vi "AlliGator Compute Sliced Mean, SDV & CV Plots.vi"(8 "error in (no error)":errorcluster, 10 "tau(I) Plot":cluster{"X Array":dbl[], "Y Array":dbl[]}, 11 "Slices Definition":T3={"Axis Start"=0.0, "Axis Stop"=0.0, "# Steps"=0, "Step Size"=1.0, "Step Definition"=enum."# Steps", "Upper Percentile"=1.0, "Lower Percentile"=1.0, "Min # Data Points/Slice"=1, "Output Abscissa Statistics Plots"=FALSE, "Bin Location"=enum."Left", "# Elements"=1, "Bootstrap CV's SDV"=FALSE, "# Replicas"=1} {"# Replicas" min=1; "# Elements" min=0; "Min # Data Points/Slice" min=0 max=100; "Lower Percentile" min=0.0 max=100.0; "Upper Percentile" min=0.0 max=100.0; "Step Size" min=1.0; "# Steps" min=1}) -> (0 "error out":errorcluster, 1 "Bootstrap CV's SDV":bool, 2 "Bin Intensity Distribution (unused)":cluster{"Intensity Array":sgl[]}[](array[cluster]), 3 "Result Plots Cluster":T1)   [LabVIEW 2021, in "AlliGator Lifetime & Other Parameters.lvlib"]
doc: "Computes sliced data statistics."
uses:
  AlliGator Lifetime & Other Parameters.lvlib
  Graphs/XY Graph/XY Graph Sliced Mean & SDV Step Definition.ctl
  AlliGator Intensity Slice Definition.ctl
  Graphs/XY Graph/XY Graph Sliced CV Abscissa Location.ctl
  Decay Fit Parameter Map/AlliGator Sliced Analysis Plots.ctl
  Graphs/XY Graph/XY Graph Plot Data.ctl
  f27c31c8-11a2-4adc-8bf5-3f0847906007.vi
  e52038b9-098e-46eb-bc49-b571e133bb6c.vi
  <userlib>/_OpenG.lib/array/array.llb/Sort 1D Array (DBL)__ogtk.vi
  <vilib>/gmath/statdist.llb/st_Percentiles (array).vi
  <vilib>/Utility/error.llb/Error Cluster From Error Code.vi
  <userlib>/_OpenG.lib/array/array.llb/openg_array.lvlib
  <vilib>/gmath/NI_Gmath.lvlib
  Error/Error.lvlib
  Graphs/XY Graph/XY Graph Add-Ons.lvlib
  Decay Fit Parameter Map/AlliGator Decay Fit Parameter Map.lvlib
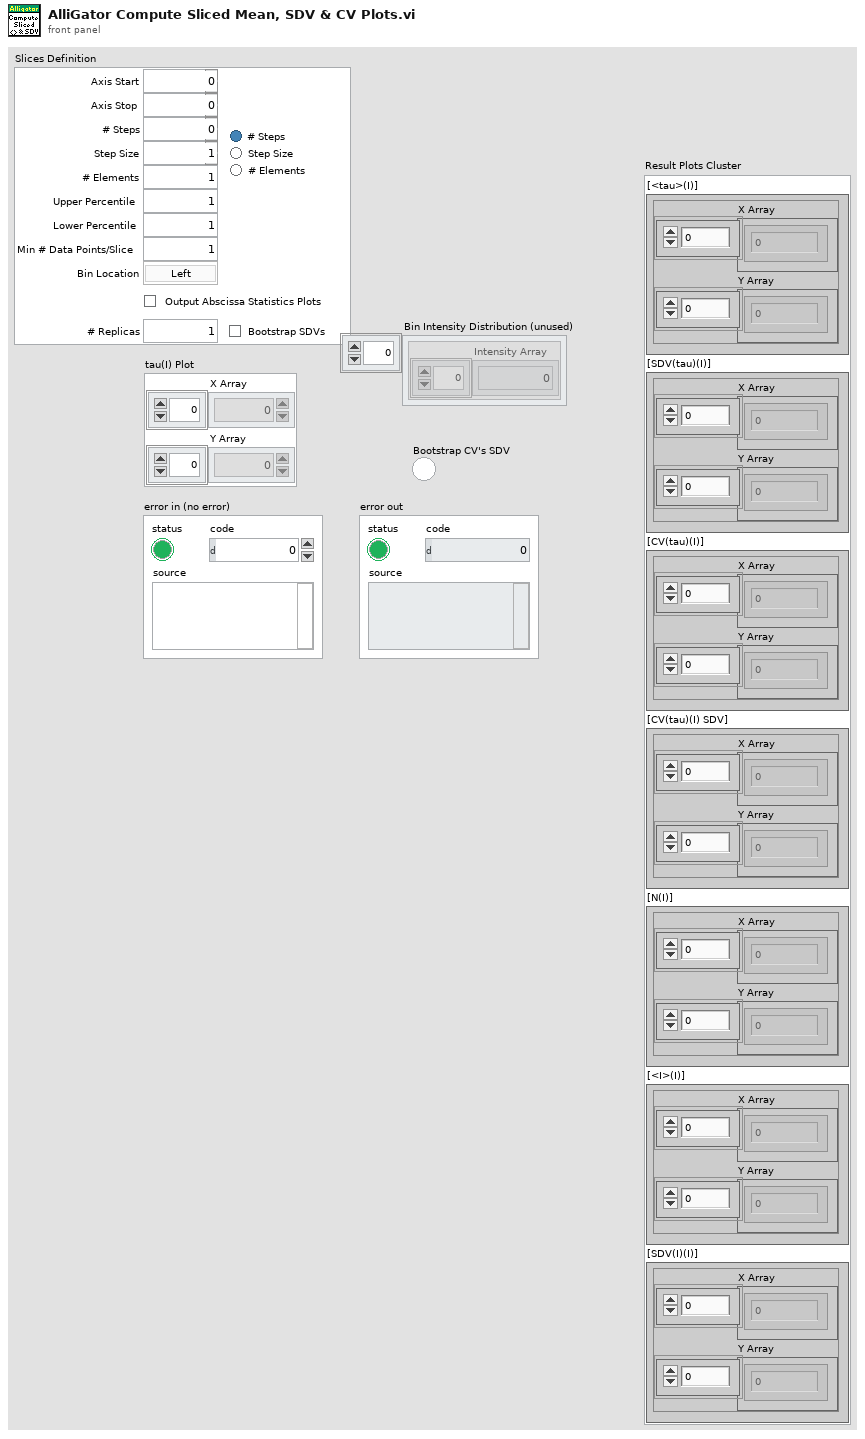
[diagram p1: front panel]
types:
  T1 = typedef "AlliGator Decay Fit Parameter Map.lvlib/AlliGator Sliced Analysis Plots.ctl" = cluster{"[<tau>(I)]":T2, "[SDV(tau)(I)]":T2, "[CV(tau)(I)]":T2, "[CV(tau)(I) SDV]":T2, "[N(I)]":T2, "[<I>(I)]":T2, "[SDV(I)(I)]":T2}
  T2 = typedef "XY Graph Add-Ons.lvlib/XY Graph Plot Data.ctl" = cluster{"X Array":dbl[], "Y Array":dbl[]}
  T3 = typedef "XY Graph Add-Ons.lvlib/XY Graph Sliced Mean & SDV Step Definition.ctl" = cluster{"Axis Start":dbl, "Axis Stop":dbl, "# Steps":i32, "Step Size":dbl, "Step Definition":T4, "Upper Percentile":dbl, "Lower Percentile":dbl, "Min # Data Points/Slice":i32, "Output Abscissa Statistics Plots":bool, "Bin Location":T5, "# Elements":i32, "Bootstrap CV's SDV":bool, "# Replicas":i32}
  T4 = typedef "AlliGator Lifetime & Other Parameters.lvlib/AlliGator Intensity Slice Definition.ctl" = enum32{"# Steps", "Step Size", "# Elements"}
  T5 = typedef "XY Graph Add-Ons.lvlib/XY Graph Sliced CV Abscissa Location.ctl" = enum16{"Left", "Center", "Mean", "Right"}
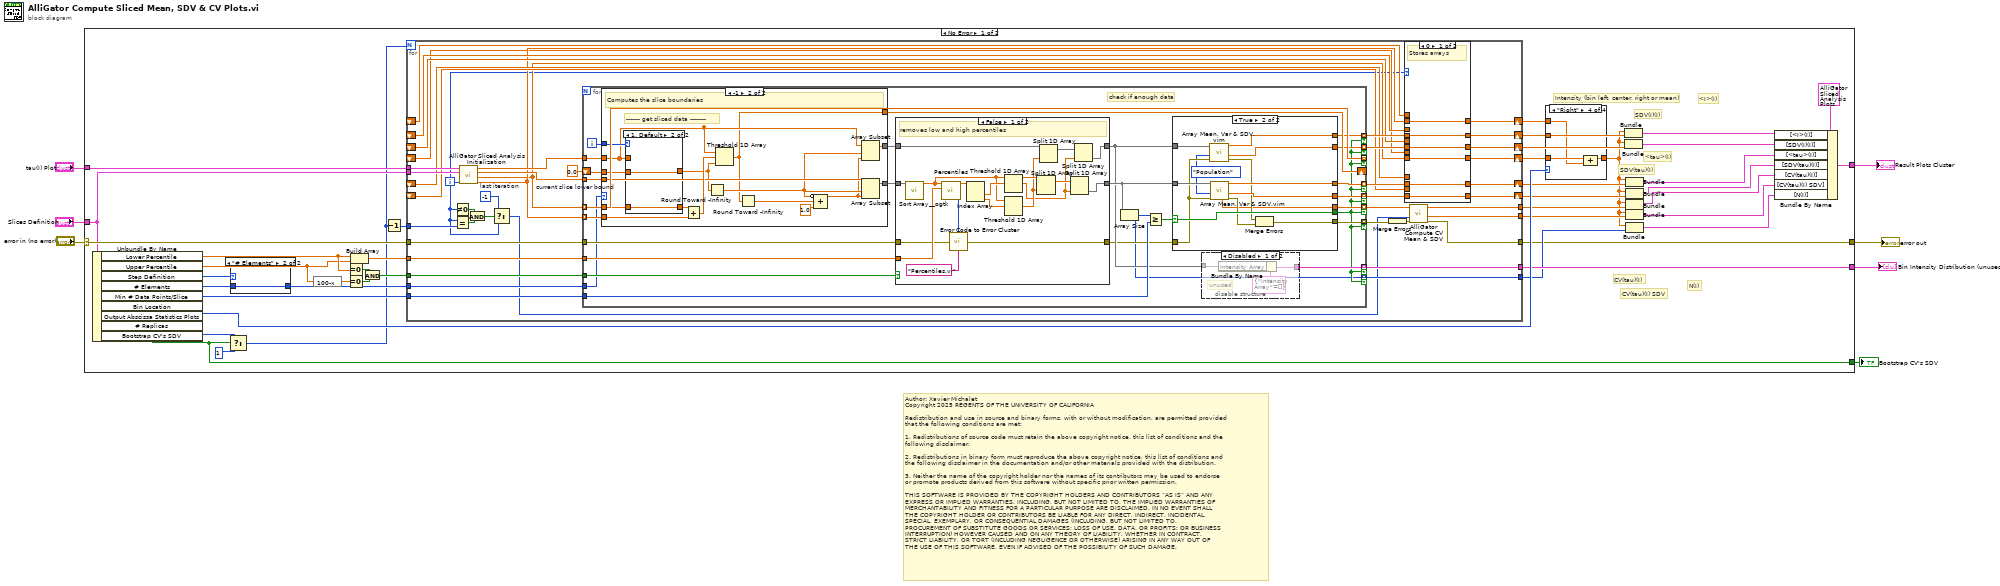
[diagram p0: block diagram]
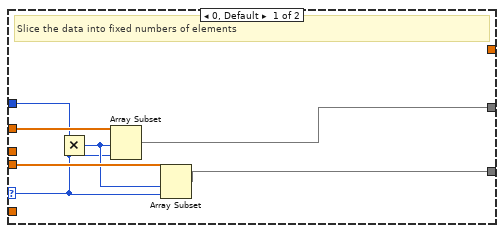
[diagram p5: hidden frame]
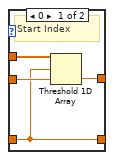
[diagram p6: hidden frame]
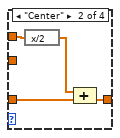
[diagram p9: hidden frame]
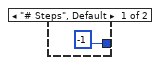
[diagram p11: hidden frame]
diagram:
  # "Author: Xavier Michalet\nCopyright 2025 REGENTS OF THE UNIVERSITY OF CALIFORNIA\n\nRedistribution and use in source and binary forms, with or without modification, are permitted provided\nthat the following conditions are met:\n\n1. Redistributions of source code must retain the above copyright notice, this list of conditions and the\nfollowing disclaimer.\n\n2. Redistributions in binary form must reproduce the above copyright notice, this list of conditions and\nthe following disclaimer in the documentation and/or other materials provided with the distribution.\n\n3. Neither the name of the copyright holder nor the names of its contributors may be used to endorse \nor promote products derived from this software without specific prior written permission.\n\nTHIS SOFTWARE IS PROVIDED BY THE COPYRIGHT HOLDERS AND CONTRIBUTORS “AS IS” AND ANY \nEXPRESS OR IMPLIED WARRANTIES, INCLUDING, BUT NOT LIMITED TO, THE IMPLIED WARRANTIES OF\nMERCHANTABILITY AND FITNESS FOR A PARTICULAR PURPOSE ARE DISCLAIMED. IN NO EVENT SHALL\nTHE COPYRIGHT HOLDER OR CONTRIBUTORS BE LIABLE FOR ANY DIRECT, INDIRECT, INCIDENTAL, \nSPECIAL, EXEMPLARY, OR CONSEQUENTIAL DAMAGES (INCLUDING, BUT NOT LIMITED TO, \nPROCUREMENT OF SUBSTITUTE GOODS OR SERVICES; LOSS OF USE, DATA, OR PROFITS; OR BUSINESS\nINTERRUPTION) HOWEVER CAUSED AND ON ANY THEORY OF LIABILITY, WHETHER IN CONTRACT, \nSTRICT LIABILITY, OR TORT (INCLUDING NEGLIGENCE OR OTHERWISE) ARISING IN ANY WAY OUT OF\nTHE USE OF THIS SOFTWARE, EVEN IF ADVISED OF THE POSSIBILITY OF SUCH DAMAGE."
  n1 = case shown="No Error" "error in (no error)" {
    selector: "error in (no error)" -> [w36 w207]
    tunnel: "tau(I) Plot" -> [w32 _]
    tunnel: "Slices Definition" -> [w31 _]
    tunnel: [w17 w207] -> w4
    tunnel: [w39 _] -> w3
    tunnel: [w12 _] -> w2
    tunnel: [w10 _] -> w1
    frame No Error {
      # "CV(tau)(I) SDV"
      # "N(I)"
      # "CV(tau)(I)"
      # "SDV(tau)(I)"
      # "<tau>(I)"
      # "SDV(I)(I)"
      # "<I>(I)"
      # "Intensity (bin left, center, right or mean)"
      n2 = Unbundle By Name(w31) -> ("Lower Percentile"=w47:dbl, "Upper Percentile"=w42:dbl, "Step Definition"=w35:T4, "# Elements"=w34:i32, "Min # Data Points/Slice"=w45:i32, "Bin Location"=w40:T5, "# Replicas"=w38:i32, "Bootstrap CV's SDV"=w12:bool)  [unwired: 1 out]
      n3 = Select(t=w38, s=w12, f=1) -> (s? t:f=w9:i32)
      n4 = case shown="\"# Elements\"" w35 {
        tunnel: w34 -> [_ w206]
        tunnel: [-1 ("# Elements") w206] -> w33
        frame "# Steps", Default {
        }
        frame "# Elements" {
        }
      }
      n5 = expression code="100-x"(w42) -> (w41:dbl)
      n6 = Equal To 0?(x=w47) -> (x = 0?=w46:bool)
      n7 = Equal To 0?(x=w41) -> (x = 0?=w44:bool)
      n8 = Build Array(w47, w42) -> (w48:dbl[])
      n9 = And(x=w46, y=w44) -> (x .and. y?=w43:bool)
      n10 = Decrement(x=w9) -> (x-1=w8:i32)
      n11 = for {
        N: w9 -> [_]
        tunnel: [w91] -> w26
        tunnel: w48 -> [w90]
        tunnel: w45 -> [w89]
        tunnel: w43 -> [w88]
        tunnel: [w62] -> w21
        tunnel: [w86] -> w39
        tunnel: [w58] -> w17
        tunnel: w36 -> [w85]
        tunnel: w33 -> [w84]
        tunnel: w32 -> [w83]
        tunnel: w31 -> [w82]
        shift-right: [w77] -> w18
        shift-left: _ -> [w66]
        shift-right: [w75] -> w24
        shift-left: _ -> [w67]
        shift-right: [w74] -> w19
        shift-left: _ -> [w56]
        shift-right: [w72] -> w30
        shift-left: _ -> [w68]
        shift-right: [w70] -> w29
        shift-left: _ -> [w69]
        shift-right: [w64] -> w16
        shift-left: _ -> [w63]
        tunnel: [w61] -> w15
        tunnel: w8 -> [w55]
        i -> [w50]
        w51 = -1  # last iteration
        w79 = 0.0  # current slice lower bound
        n12 = Not Equal To 0?(x=w50) -> (x != 0?=w54:bool)
        n13 = Equal?(x=w50, y=w55) -> (x = y?=w53:bool)
        n14 = call "AlliGator Sliced Analysis Initialization.vi"("Iteration (0)"=w50, "Slices Definition"=w82, "tau(I) Plot"=w83) -> ("[delta I_i]"=w65:dbl[], "[I_i]"=w57:dbl[], "[tau]"=w80:dbl[], "Sorted [I]"=w81:dbl[])  [unwired: 4 in, 1 out]
        n15 = And(x=w54, y=w53) -> (x .and. y?=w52:bool)
        n16 = Select(t=w51, s=w52, f=w50) -> (s? t:f=w49:i32)
        n17 = for {
          tunnel: w57 -> [w121] mode=indexing
          tunnel: w81 -> [w117]
          tunnel: w80 -> [w127]
          shift-right: [w115] -> _
          shift-left: w79 -> [w129]
          tunnel: w65 -> [w128] mode=indexing
          tunnel: [w126] -> w73 mode=indexing if=w107
          tunnel: [w125] -> w71 mode=indexing if=w107
          tunnel: [w104] -> w91 mode=indexing if=w107
          tunnel: w90 -> [w124]
          tunnel: w89 -> [w122]
          tunnel: [w121] -> _ mode=indexing if=w107
          tunnel: w88 -> [w118]
          tunnel: [w114] -> w78 mode=indexing if=w107
          tunnel: [w113] -> w76 mode=indexing if=w107
          tunnel: [w112] -> w87 mode=indexing if=w107
          tunnel: [w110] -> w86 mode=indexing if=w107
          tunnel: [w108] -> w60 mode=indexing if=w107
          tunnel: w85 -> [w106]
          tunnel: w84 -> [w105]
          i -> [w130]
          # "check if enough data"
          n18 = case shown="-1" w105 {
            selector: w105 -> [w165 _]
            tunnel: w130 -> [w169 w186]
            tunnel: w129 -> [_ w185]
            tunnel: w128 -> [_ w183]
            tunnel: w127 -> [w167 w181]
            tunnel: w121 -> [_ w177]
            tunnel: [w164 w176] -> w119
            tunnel: w117 -> [w170 w175]
            tunnel: [w168 w172] -> w116
            tunnel: [_ w171] -> w115
            frame 0, Default {
              # "Slice the data into fixed numbers of elements"
              n19 = Multiply(x=w169, y=w165) -> (x*y=w166:i32)
              n20 = Array Subset(array=w170, index=w166, length=w165) -> (w168:dbl[])
              n21 = Array Subset(array=w167, index=w166, length=w165) -> (w164:dbl[])
            }
            frame -1 {
              # "------- get sliced data --------"
              # "Computes the slice boundaries"
              n22 = case shown="1, Default" w186 {
                tunnel: w175 -> [w190 _]
                tunnel: w177 -> [w187 w192]
                tunnel: w185 -> [w189 w191]
                tunnel: [w188 w191] -> w180
                tunnel: [w187 w192] -> w184
                frame 0 {
                  # "Start Index"
                  n23 = Threshold 1D Array(1:w189, 2:w187, 3:w190) -> (0:w188:dbl)
                }
                frame 1, Default {
                }
              }
              n24 = Add(x=w184, y=w183) -> (x+y=w182:dbl)
              n25 = Round Toward -Infinity(1:w180) -> (0:w174:dbl)
              n26 = Threshold 1D Array(1:w180, 2:w182, 3:w175) -> (0:w171:dbl)
              n27 = Round Toward -Infinity(1:w171) -> (0:w179:dbl)
              n28 = Compound Arithmetic op=ADD(invert w174, w179, 1.0 ("value")) -> (w173:dbl)
              n29 = Array Subset(array=w175, index=w174, length=w173) -> (w172:dbl[])
              n30 = Array Subset(array=w181, index=w174, length=w173) -> (w176:dbl[])
            }
          }
          n31 = case shown="False" w118 {
            tunnel: w124 -> [w161 _]
            tunnel: [w159 w163] -> w123
            tunnel: w119 -> [w155 w163]
            tunnel: w116 -> [w153 w162]
            tunnel: [w150 w162] -> w111
            tunnel: [w146 _] -> w109
            tunnel: w106 -> [w145 _]
            frame False {
              # "removes low and high percentiles"
              n32 = call-poly <userlib>:"Sort Array__ogtk.vi"("Array in"=w155) -> ("Sorted Array out"=w154:dbl[])  [unwired: 9 in, 1 out]
              n33 = call-poly <vilib>:"Percentiles.vi"("p array"=w161, "x array"=w154) -> ("error"=w148:i32, "percentiles"=w160:dbl[])  [unwired: 8 in]
              n34 = call "Error Code to Error Cluster.vi"("Error Code"=w148, "Error Source"="Percentiles.vi", "Error In"=w145) -> ("Error Out"=w146:errorcluster)  [unwired: 12 in]
              n35 = Index Array(array=w160) -> (element #1=w158:dbl, element #2=w156:dbl)  [unwired: 2 in]
              n36 = Threshold 1D Array(2:w158, 3:w154) -> (0:w149:dbl)  [unwired: 1 in]
              n37 = Threshold 1D Array(2:w156, 3:w154) -> (0:w152:dbl)  [unwired: 1 in]
              n38 = Split 1D Array(array=w154, index=w152) -> (first subarray=w157:dbl[])  [unwired: 1 out]
              n39 = Split 1D Array(array=w153, index=w152) -> (first subarray=w151:dbl[])  [unwired: 1 out]
              n40 = Split 1D Array(array=w157, index=w149) -> (second subarray=w159:dbl[])  [unwired: 1 out]
              n41 = Split 1D Array(array=w151, index=w149) -> (second subarray=w150:dbl[])  [unwired: 1 out]
            }
            frame True {
              # "Do not reject outliers"
            }
          }
          n42 = Array Size(array=w123) -> (size(s)=w104:i32)
          n43 = Greater Or Equal?(x=w104, y=w122) -> (x >= y?=w120:bool)
          n44 = case shown="True" w120 {
            selector: w120 -> [_ w141]
            tunnel: [_ w144] -> w126
            tunnel: [_ w143] -> w125
            tunnel: w123 -> [_ w142]
            tunnel: [_ w141] -> w107
            tunnel: w111 -> [_ w140]
            tunnel: [_ w139] -> w114
            tunnel: [_ w138] -> w113
            tunnel: [_ w133] -> w112
            tunnel: w109 -> [w131 w137]
            tunnel: [w131 w134] -> w108
            frame False {
              # "Not enough data"
            }
            frame True {
              w132 = enum16{"Sample", "Population"}."Population" ("Weighting (Sample)")
              n45 = call "Array Mean, Var & SDV.vim"("Error In"=w137, "Weighting (Sample)"=w132, "Array"=w140) -> ("Error Out"=w135:errorcluster, "Array SDV"=w138:dbl, "Array Mean"=w139:dbl)  [unwired: 3 in, 3 out]
              n46 = call "Array Mean, Var & SDV.vim"("Error In"=w137, "Weighting (Sample)"=w132, "Array"=w142) -> ("Error Out"=w136:errorcluster, "Array SDV"=w143:dbl, "Array Mean"=w144:dbl, "Array CV"=w133:dbl)  [unwired: 3 in, 2 out]
              n47 = Merge Errors(w135, w136) -> (w134:errorcluster)
            }
          }
          n48 = disable-structure shown="Disabled" {
            disable-tunnel: w111 -> [w194 _]
            disable-tunnel: [w193 _] -> w110
            frame Disabled {
              # "unused"
              n49 = Bundle By Name(cluster=cluster{"Intensity Array":sgl[]} {"Intensity Array"=[]} ("Cluster"), "Intensity Array"=w194) -> (w193:cluster{"Intensity Array":sgl[]})
            }
            frame Enabled {
            }
          }
        }
        n50 = Merge Errors(w60) -> (w59:errorcluster)
        n51 = case shown="0" w50 {
          tunnel: w78 -> [w97 _]
          tunnel: [w97 w99] -> w77
          tunnel: w76 -> [w96 _]
          tunnel: [w96 w100] -> w75
          tunnel: w57 -> [w95 _]
          tunnel: [w95 w101] -> w74
          tunnel: w73 -> [w94 _]
          tunnel: [w94 w102] -> w72
          tunnel: w71 -> [w93 _]
          tunnel: [w93 w103] -> w70
          tunnel: w69 -> [_ w103]
          tunnel: w68 -> [_ w102]
          tunnel: w56 -> [_ w101]
          tunnel: w67 -> [_ w100]
          tunnel: w66 -> [_ w99]
          tunnel: w65 -> [w92 _]
          tunnel: [w92 w98] -> w64
          tunnel: w63 -> [_ w98]
          frame 0 {
            # "Stores arrays"
          }
          frame 1, Default {
            # "Pass stored arrays"
          }
        }
        n52 = call "AlliGator Compute CV Mean & SDV.vi"("Error In"=w59, "Iteration"=w49, "CV Array in"=w87) -> ("Error Out"=w58:errorcluster, "CV SDV Array"=w61:dbl[], "Average CV Array"=w62:dbl[])  [unwired: 6 in]
      }
      n53 = case shown="\"Right\"" w40 {
        tunnel: w19 -> [w196 w200 _ w204]
        tunnel: [w196 w198 w201 w203] -> w14
        tunnel: w16 -> [_ w199 _ w202]
        tunnel: w18 -> [_ _ w201 _]
        frame "Left", Default {
        }
        frame "Center" {
          n54 = expression code="x/2"(w199) -> (w197:dbl[])
          n55 = Compound Arithmetic op=ADD(w197, w200) -> (w198:dbl[])
        }
        frame "Mean" {
        }
        frame "Right" {
          n56 = Compound Arithmetic op=ADD(w204, w202) -> (w203:dbl[])
        }
      }
      n57 = Bundle("[I_i]"=w14, w18) -> (w23:cluster{"[I_i]":dbl[], dbl[]})  [unwired: 1 in]
      n58 = Bundle("[I_i]"=w14, w24) -> (w22:cluster{"[I_i]":dbl[], dbl[]})  [unwired: 1 in]
      n59 = Bundle("[I_i]"=w14, w30) -> (w28:cluster{"[I_i]":dbl[], dbl[]})  [unwired: 1 in]
      n60 = Bundle("[I_i]"=w14, w29) -> (w27:cluster{"[I_i]":dbl[], dbl[]})  [unwired: 1 in]
      n61 = Bundle("[I_i]"=w14, "Average CV Array"=w21) -> (w20:cluster{"[I_i]":dbl[], "Average CV Array":dbl[]})  [unwired: 1 in]
      n62 = Bundle("[I_i]"=w14, "CV SDV Array"=w15) -> (w13:cluster{"[I_i]":dbl[], "CV SDV Array":dbl[]})  [unwired: 1 in]
      n63 = Bundle("[I_i]"=w14, w26) -> (w25:cluster{"[I_i]":dbl[], i32[]})  [unwired: 1 in]
      n64 = Bundle By Name(cluster=T1 {"[<tau>(I)]"={"X Array"=[], "Y Array"=[]}, "[SDV(tau)(I)]"={"X Array"=[], "Y Array"=[]}, "[CV(tau)(I)]"={"X Array"=[], "Y Array"=[]}, "[CV(tau)(I) SDV]"={"X Array"=[], "Y Array"=[]}, "[N(I)]"={"X Array"=[], "Y Array"=[]}, "[<I>(I)]"={"X Array"=[], "Y Array"=[]}, "[SDV(I)(I)]"={"X Array"=[], "Y Array"=[]}} ("Result Plots Cluster"), "[<I>(I)]"=w23, "[SDV(I)(I)]"=w22, "[<tau>(I)]"=w28, "[SDV(tau)(I)]"=w27, "[CV(tau)(I)]"=w20, "[CV(tau)(I) SDV]"=w13, "[N(I)]"=w25) -> (w10:T1)
    }
    frame Error {
    }
  }
  "error out" <- w4
  "Bin Intensity Distribution (unused)" <- w3
  "Bootstrap CV's SDV" <- w2
  "Result Plots Cluster" <- w1
